vi "Injection Command Plot - EPT.vi"(9 "System":T6={"Battery [V]"=13.7, "Engine Speed [RPM]"=1000.0, "Rotations"=1, "Injector Configuration"={"Resistance [Ohm]"=1.0, "Inductance [Henery]"=0.001, "Capacitance [Farad]"=5e-06}, "Description"=""} {"Injector Configuration"."Capacitance [Farad]" format="%#_6p"; "Injector Configuration"."Inductance [Henery]" format="%#_6p"; "Injector Configuration"."Resistance [Ohm]" format="%#_6p"; "Rotations" min=1 max=2; "Engine Speed [RPM]" min=500 max=50000; "Battery [V]" min=6 max=48}, 10 "Injection Command":T1={"Mode"=enum."Off", "Digital Input"=enum."Unused", "Default Profile Index"=0, "Cal Freq [Hz]"=0.0, "Cal Duration [s]"=0.0, "Cal Increment [s]"=0.0, "Cal Pulses"=0, "TMP Command Sequence"=[{"Duration [s]"=0.0, "Level"=FALSE, "Run/Stop"=FALSE, "Profile Index"=0}, {"Duration [s]"=0.0, "Level"=FALSE, "Run/Stop"=FALSE, "Profile Index"=0}, {"Duration [s]"=0.0, "Level"=FALSE, "Run/Stop"=FALSE, "Profile Index"=0}, {"Duration [s]"=0.0, "Level"=FALSE, "Run/Stop"=FALSE, "Profile Index"=0}, {"Duration [s]"=0.0, "Level"=FALSE, "Run/Stop"=FALSE, "Profile Index"=0}, {"Duration [s]"=0.0, "Level"=FALSE, "Run/Stop"=FALSE, "Profile Index"=0}, {"Duration [s]"=0.0, "Level"=FALSE, "Run/Stop"=FALSE, "Profile Index"=0}, {"Duration [s]"=0.0, "Level"=FALSE, "Run/Stop"=FALSE, "Profile Index"=0}], "EPT TDC Offset [CAD]"=0.0, "EPT Window Start [DBTDC]"=0.0, "EPT Window End [DBTDC]"=0.0, "EPT Angles"=[{"Enable"=FALSE, "Timing [DBTDC]"=0.0, "Duration [s]"=0.0, "Profile Index"=0}, {"Enable"=FALSE, "Timing [DBTDC]"=0.0, "Duration [s]"=0.0, "Profile Index"=0}, {"Enable"=FALSE, "Timing [DBTDC]"=0.0, "Duration [s]"=0.0, "Profile Index"=0}, {"Enable"=FALSE, "Timing [DBTDC]"=0.0, "Duration [s]"=0.0, "Profile Index"=0}, {"Enable"=FALSE, "Timing [DBTDC]"=0.0, "Duration [s]"=0.0, "Profile Index"=0}, {"Enable"=FALSE, "Timing [DBTDC]"=0.0, "Duration [s]"=0.0, "Profile Index"=0}, {"Enable"=FALSE, "Timing [DBTDC]"=0.0, "Duration [s]"=0.0, "Profile Index"=0}, {"Enable"=FALSE, "Timing [DBTDC]"=0.0, "Duration [s]"=0.0, "Profile Index"=0}], "EPT Skip Fire"=FALSE, "EPT Skip Index"=0, "EPT Precharge Duration [s]"=0.0, "EPT Precharge Profile Index"=0} {"EPT Precharge Profile Index" max=15; "EPT Precharge Duration [s]" min=0 format="%#_4p"; "Default Profile Index" max=15; "Cal Increment [s]" format="%#_3p"; "TMP Command Sequence"."Profile Index" max=7; "TMP Command Sequence"."Duration [s]" min=0 max=100 format="%#_3p"; "Cal Pulses" max=511; "EPT Skip Index" max=7; "EPT Angles"."Profile Index" max=7; "EPT Angles"."Duration [s]" min=0 max=100 format="%#_3p"; "Cal Duration [s]" format="%#_3p"; "Cal Freq [Hz]" format="%#_3p"}) -> (2 "Plot":cluster{"Array":sgl[], "Array":sgl[]}[](array[cluster]))   [LabVIEW 2016]
uses:
  <vilib>/Powertrain Controls/Device Drivers/DCM/Rev0/UI/System Configuration.ctl
  <vilib>/Powertrain Controls/Device Drivers/DCM/Rev0/UI/Injector Configuration.ctl
  <vilib>/Powertrain Controls/Device Drivers/DCM/DI/RT/Command.ctl
  <vilib>/Powertrain Controls/Device Drivers/DCM/DI/FPGA/Mode.ctl
  <vilib>/Powertrain Controls/Device Drivers/DCM/Rev0/FPGA/Digital Channel.ctl
  <vilib>/Powertrain Controls/Device Drivers/DCM/DI/RT/Command Sequence.ctl
  <vilib>/Powertrain Controls/Device Drivers/DCM/DI/RT/Angle Control.ctl
  <vilib>/Powertrain Controls/Device Drivers/DCM/Rev0/UI/DCM - UI.lvlib
  <vilib>/Powertrain Controls/Device Drivers/DCM/DI/FPGA/DCM - FPGA - DI.lvlib
  <vilib>/Powertrain Controls/Device Drivers/DCM/Rev0/FPGA/DCM - FPGA.lvlib
  <vilib>/Powertrain Controls/Device Drivers/DCM/DI/RT/DCM - RT - DI.lvlib
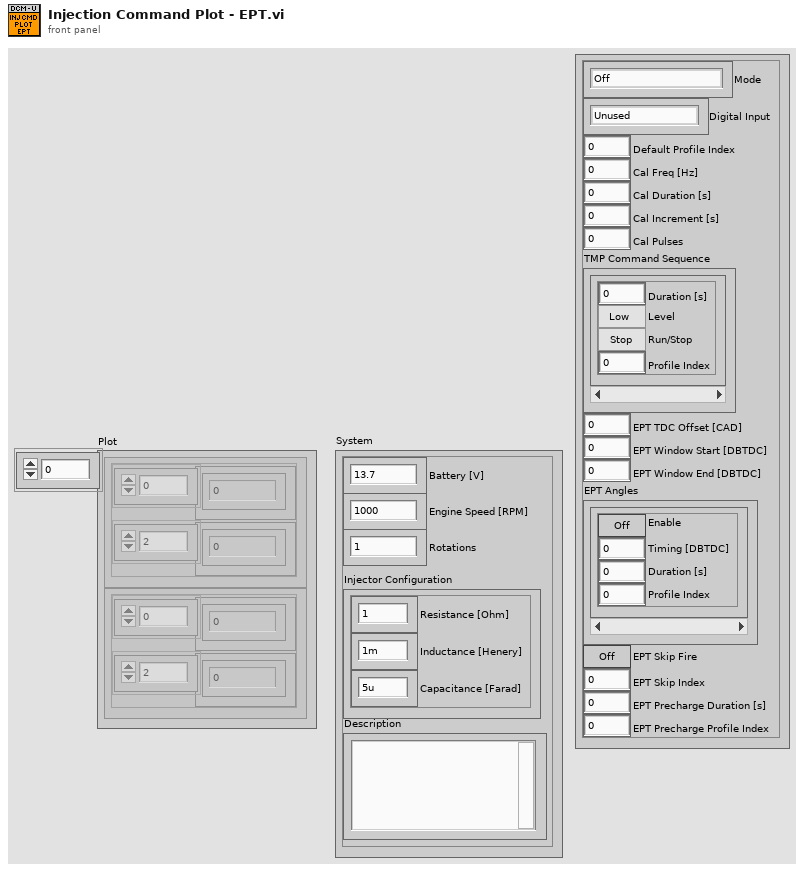
[diagram p1: front panel]
types:
  T1 = typedef "DCM - RT - DI.lvlib/Command.ctl" = cluster{"Mode":T2, "Digital Input":T3, "Default Profile Index":u8, "Cal Freq [Hz]":sgl, "Cal Duration [s]":sgl, "Cal Increment [s]":sgl, "Cal Pulses":u16, "TMP Command Sequence":T4[], "EPT TDC Offset [CAD]":sgl, "EPT Window Start [DBTDC]":sgl, "EPT Window End [DBTDC]":sgl, "EPT Angles":T5[], "EPT Skip Fire":bool, "EPT Skip Index":u8, "EPT Precharge Duration [s]":sgl, "EPT Precharge Profile Index":u8}
  T2 = typedef "DCM - FPGA - DI.lvlib/Mode.ctl" = enum8{"Off", "Direct", "Calibration", "Triggered Multi-Pulse", "Engine Position Tracking"}
  T3 = typedef "DCM - FPGA.lvlib/Digital Channel.ctl" = enum8{"Unused", "User OS", "Diff IO 1", "Diff IO 2", "Diff IO 3", "Diff IO 4", "Diff IO 5", "Diff IO 6", "Diff IO 7", "Diff IO 8", "Aux 1", "Aux 2", "Aux 3", "Aux 4", "Aux 5", "Aux 6", "Aux 7", "Aux 8", "Aux 9", "Aux 10", "Aux 11", "Aux 12", "Aux 13", "Aux 14", "Aux 15", "Aux 16"}
  T4 = typedef "DCM - RT - DI.lvlib/Command Sequence.ctl" = cluster{"Duration [s]":sgl, "Level":bool, "Run/Stop":bool, "Profile Index":u8}
  T5 = typedef "DCM - RT - DI.lvlib/Angle Control.ctl" = cluster{"Enable":bool, "Timing [DBTDC]":sgl, "Duration [s]":sgl, "Profile Index":u8}
  T6 = typedef "DCM - UI.lvlib/System Configuration.ctl" = cluster{"Battery [V]":sgl, "Engine Speed [RPM]":sgl, "Rotations":u8, "Injector Configuration":T7, "Description":string}
  T7 = typedef "DCM - UI.lvlib/Injector Configuration.ctl" = cluster{"Resistance [Ohm]":sgl, "Inductance [Henery]":sgl, "Capacitance [Farad]":sgl}
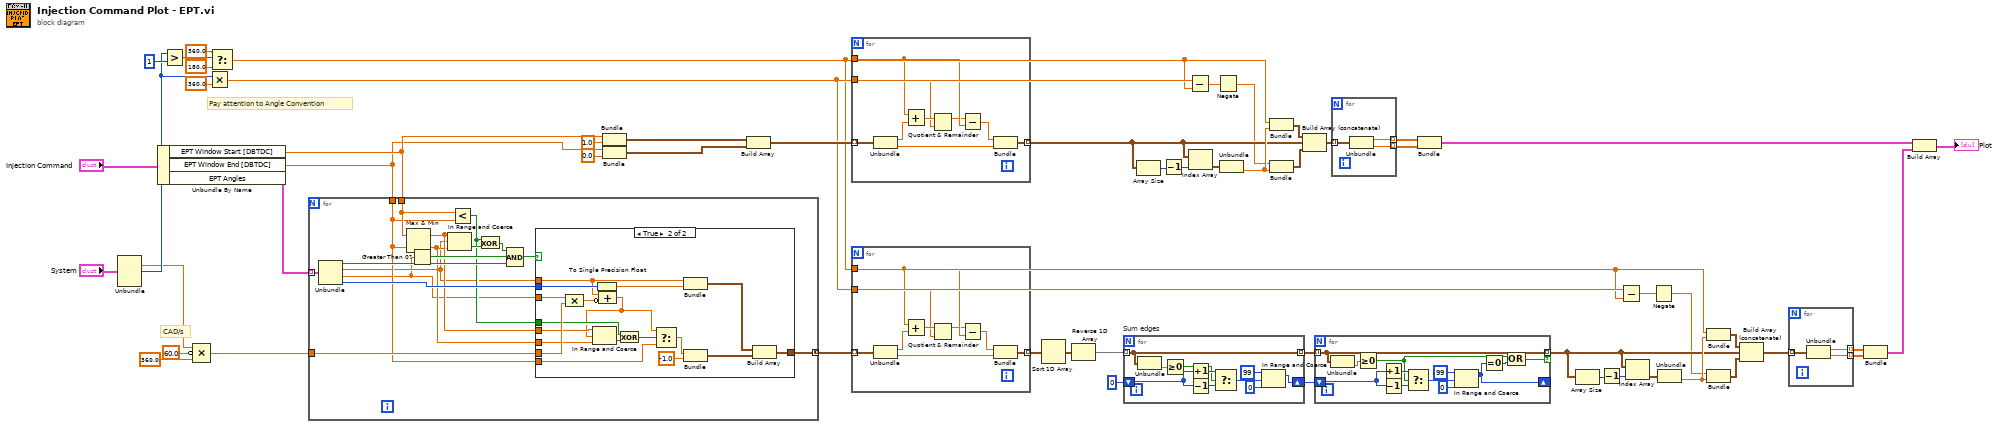
[diagram p0: block diagram]
diagram:
  # "Pay attention to Angle Convention"
  # "CAD/s"
  n1 = Unbundle("System") -> ("Engine Speed [RPM]"=w30:sgl, "Rotations"=w31:u8)  [unwired: 3 out]
  n2 = Unbundle By Name("Injection Command") -> ("EPT Window Start [DBTDC]"=w18:sgl, "EPT Window End [DBTDC]"=w17:sgl, "EPT Angles"=w19:T5[])
  n3 = Greater?(x=w31, y=u8 1) -> (0:w50:bool)
  n4 = Compound Arithmetic op=MULTIPLY(w30, invert sgl 60.0 ("value"), sgl 360.0 ("value")) -> (w5:sgl)
  n5 = Multiply(x=w31, y=sgl 360.0) -> (x*y=w34:sgl)
  n6 = Select(t=sgl 360.0 ("y"), s=w50, f=sgl 180.0 ("y")) -> (s? t:f=w9:sgl)
  n7 = for {
    tunnel: [w72] -> w32 mode=concatenating
    tunnel: w5 -> [w71]
    tunnel: w19 -> [w70] mode=indexing
    tunnel: w18 -> [w62]
    tunnel: w17 -> [w59]
    n8 = Unbundle(w70) -> ("Enable"=w67:bool, "Timing [DBTDC]"=w58:sgl, "Duration [s]"=w57:sgl, "Profile Index"=w69:u8)
    n9 = Max & Min(x=w62, y=w59) -> (max(x,y)=w61:sgl, min(x,y)=w60:sgl)
    n10 = Greater Than 0?(x=w57) -> (x > 0?=w68:bool)
    n11 = In Range and Coerce(upper limit=w61, x=w58, lower limit=w60) -> (In Range?=w64:bool)  [unwired: 1 out]
    n12 = Less?(x=w62, y=w59) -> (x < y?=w63:bool)
    n13 = Exclusive Or(1:w64, 2:w63) -> (0:w65:bool)
    n14 = Compound Arithmetic op=AND(w65, w68, w67) -> (w66:bool)
    n15 = case shown="True" w66 {
      tunnel: [_ w90] -> w72
      tunnel: w58 -> [_ w83]
      tunnel: w57 -> [_ w85]
      tunnel: w69 -> [_ w89]
      tunnel: w71 -> [_ w81]
      tunnel: w63 -> [_ w79]
      tunnel: w60 -> [_ w78]
      tunnel: w61 -> [_ w77]
      tunnel: w59 -> [_ w74]
      frame False {
      }
      frame True {
        n16 = Compound Arithmetic op=MULTIPLY(w85, w81) -> (w86:sgl)
        n17 = To Single Precision Float(number=w89) -> (single precision float=w88:sgl)
        n18 = Compound Arithmetic op=ADD(w83, invert w86) -> (w75:sgl)
        n19 = In Range and Coerce(upper limit=w77, x=w75, lower limit=w78) -> (In Range?=w80:bool)  [unwired: 1 out]
        n20 = Exclusive Or(1:w80, 2:w79) -> (0:w76:bool)
        n21 = Select(t=w75, s=w76, f=w74) -> (s? t:f=w73:sgl)
        n22 = Bundle("Timing [DBTDC]"=w83, w88) -> (w82:cluster{"Timing [DBTDC]":sgl, sgl})  [unwired: 1 in]
        n23 = Bundle("EPT Window End [DBTDC]"=w73, sgl -1.0) -> (w84:cluster{"EPT Window End [DBTDC]":sgl, sgl})  [unwired: 1 in]
        n24 = Build Array(w82, w84) -> (w90:cluster{"EPT Window End [DBTDC]":sgl, sgl}[])
      }
    }
  }
  n25 = Bundle("EPT Window Start [DBTDC]"=w18, "y"=sgl 1.0) -> (w21:cluster{"EPT Window Start [DBTDC]":sgl, "y":sgl})  [unwired: 1 in]
  n26 = Bundle("EPT Window End [DBTDC]"=w17, "y"=sgl 0.0) -> (w20:cluster{"EPT Window End [DBTDC]":sgl, "y":sgl})  [unwired: 1 in]
  n27 = Build Array(w21, w20) -> (w46:cluster{"EPT Window End [DBTDC]":sgl, "y":sgl}[])
  n28 = for {
    tunnel: w46 -> [w99] mode=indexing
    tunnel: w9 -> [w94]
    tunnel: w34 -> [w95]
    tunnel: [w93] -> w13 mode=indexing
    n29 = Unbundle(w99) -> ("EPT Window End [DBTDC]"=w97:sgl, "y"=w98:sgl)
    n30 = Add(x=w94, y=w97) -> (x+y=w96:sgl)
    n31 = Quotient & Remainder(x=w96, y=w95) -> (x-y*floor(x/y)=w92:sgl)  [unwired: 1 out]
    n32 = Subtract(x=w92, y=w94) -> (x-y=w91:sgl)
    n33 = Bundle(w91, "y"=w98) -> (w93:cluster{sgl, "y":sgl})  [unwired: 1 in]
  }
  n34 = for {
    tunnel: w32 -> [w108] mode=indexing
    tunnel: w9 -> [w103]
    tunnel: w34 -> [w104]
    tunnel: [w101] -> w14 mode=indexing
    n35 = Unbundle(w108) -> ("EPT Window End [DBTDC]"=w106:sgl, w107:sgl)
    n36 = Add(x=w103, y=w106) -> (x+y=w105:sgl)
    n37 = Quotient & Remainder(x=w105, y=w104) -> (x-y*floor(x/y)=w100:sgl)  [unwired: 1 out]
    n38 = Subtract(x=w100, y=w103) -> (x-y=w102:sgl)
    n39 = Bundle(w102, w107) -> (w101:cluster{sgl, sgl})  [unwired: 1 in]
  }
  n40 = Sort 1D Array(array=w14) -> (sorted array=w7:cluster{sgl, sgl}[])
  n41 = Reverse 1D Array(array=w7) -> (reversed array=w6:cluster{sgl, sgl}[])
  n42 = for "Sum edges" {
    tunnel: w6 -> [w114] mode=indexing
    tunnel: [w114] -> w3 mode=indexing
    shift-right: [w110] -> w2
    shift-left: 0 -> [w117]
    n43 = Unbundle(w114) -> (w118:sgl)  [unwired: 1 out]
    n44 = Greater Or Equal To 0?(x=w118) -> (x >= 0?=w109:bool)
    n45 = Increment(x=w117) -> (x+1=w115:i32)
    n46 = Decrement(x=w117) -> (x-1=w116:i32)
    n47 = Select(t=w115, s=w109, f=w116) -> (s? t:f=w113:i32)
    n48 = In Range and Coerce(upper limit=99, x=w113, lower limit=0) -> (coerced(x)=w110:i32)  [unwired: 1 out]
  }
  n49 = Array Size(array=w13) -> (size(s)=w27:i32)
  n50 = Decrement(x=w27) -> (x-1=w26:i32)
  n51 = Subtract(x=w34, y=w9) -> (x-y=w12:sgl)
  n52 = Index Array(array=w13, index=w26) -> (element=w41:cluster{sgl, "y":sgl})
  n53 = Negate(x=w12) -> (-x=w8:sgl)
  n54 = Unbundle(w41) -> ("y"=w40:sgl)  [unwired: 1 out]
  n55 = Bundle("y"=w9, "y"=w40) -> (w44:cluster{"y":sgl, "y":sgl})  [unwired: 1 in]
  n56 = Bundle(w8, "y"=w40) -> (w43:cluster{sgl, "y":sgl})  [unwired: 1 in]
  n57 = Build Array (concatenate)(w44, w13, w43) -> (w42:cluster{"y":sgl, "y":sgl}[])
  n58 = for {
    tunnel: w3 -> [w126] mode=indexing
    tunnel: [w126] -> w24 mode=indexing if=w119
    shift-right: [w122] -> _
    shift-left: w2 -> [w129]
    n59 = Unbundle(w126) -> (w130:sgl)  [unwired: 1 out]
    n60 = Greater Or Equal To 0?(x=w130) -> (x >= 0?=w120:bool)
    n61 = Increment(x=w129) -> (x+1=w127:i32)
    n62 = Decrement(x=w129) -> (x-1=w128:i32)
    n63 = Select(t=w127, s=w120, f=w128) -> (s? t:f=w125:i32)
    n64 = In Range and Coerce(upper limit=99, x=w125, lower limit=0) -> (coerced(x)=w122:i32)  [unwired: 1 out]
    n65 = Equal To 0?(x=w122) -> (x = 0?=w121:bool)
    n66 = Compound Arithmetic op=OR(w120, w121) -> (w119:bool)
  }
  n67 = for {
    tunnel: w42 -> [w133] mode=indexing
    tunnel: [w132] -> w11 mode=indexing
    tunnel: [w131] -> w10 mode=indexing
    n68 = Unbundle(w133) -> ("y"=w132:sgl, "y"=w131:sgl)
  }
  n69 = Bundle(w11, w10) -> (w45:cluster{sgl[], sgl[]})  [unwired: 1 in]
  n70 = Array Size(array=w24) -> (size(s)=w29:i32)
  n71 = Decrement(x=w29) -> (x-1=w28:i32)
  n72 = Subtract(x=w34, y=w9) -> (x-y=w16:sgl)
  n73 = Index Array(array=w24, index=w28) -> (element=w38:cluster{sgl, sgl})
  n74 = Negate(x=w16) -> (-x=w15:sgl)
  n75 = Unbundle(w38) -> (w39:sgl)  [unwired: 1 out]
  n76 = Bundle("y"=w9, w39) -> (w37:cluster{"y":sgl, sgl})  [unwired: 1 in]
  n77 = Bundle(w15, w39) -> (w4:cluster{sgl, sgl})  [unwired: 1 in]
  n78 = Build Array (concatenate)(w37, w24, w4) -> (w25:cluster{"y":sgl, sgl}[])
  n79 = for {
    tunnel: w25 -> [w136] mode=indexing
    tunnel: [w135] -> w35 mode=indexing
    tunnel: [w134] -> w36 mode=indexing
    n80 = Unbundle(w136) -> ("y"=w135:sgl, w134:sgl)
  }
  n81 = Bundle(w35, w36) -> (w33:cluster{sgl[], sgl[]})  [unwired: 1 in]
  n82 = Build Array(w45, w33) -> (→"Plot":cluster{sgl[], sgl[]}[])
